vi "Variant To Control Reference.vi"(4 "Registry Variant Accessor in":refnum<class "CConfig Variant Accessor.lvclass">, 7 "Ctl Refnum":refnum<vi>, 8 "error in (no error)":errorcluster, 9 "Value":variant, 10 "Signalling? [F]":bool, 11 "Carya Config in":refnum<class "Carya Config.lvclass">) -> (0 "error out":errorcluster, 3 "Carya Config out":refnum<class "Carya Config.lvclass">)   [LabVIEW 2013, in "Carya Config.lvclass"]
doc: "Copyright 2018, Carya Automatisering, Wiebe Walstra."
uses:
  Carya Config.lvclass
  CConfig Variant Accessor/CConfig Variant Accessor.lvclass
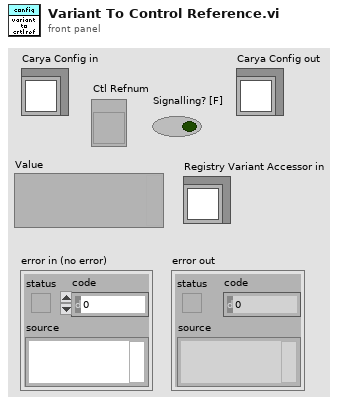
[diagram p1: front panel]
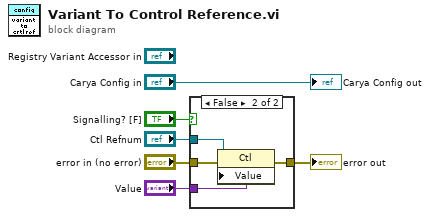
[diagram p0: block diagram]
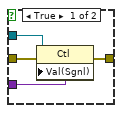
[diagram p2: hidden frame]
diagram:
  n1 = case shown="False" "Signalling? [F]" {
    tunnel: "error in (no error)" -> [w10 w14]
    tunnel: [w9 w13] -> w5
    tunnel: "Ctl Refnum" -> [w8 w12]
    tunnel: "Value" -> [w7 w11]
    frame True {
      n2 = property class="Ctl"(reference=w8, error in=w10, "Val(Sgnl)"=w7) -> (error out=w9:errorcluster)  [unwired: 1 out]
    }
    frame False {
      n3 = property class="Ctl"(reference=w12, error in=w14, "Value"=w11) -> (error out=w13:errorcluster)  [unwired: 1 out]
    }
  }
  "error out" <- w5
  "Carya Config out" <- "Carya Config in"
